vi "Checksum (SubVI).vi"(0 "StrIn":string="GPRMC,155547.000,A,0253.0515,S,07900.7371,W,0.00,,010113,,,A") -> (1 "Checksum":string, 2 "ChkSum":u8 format="%x")   [LabVIEW 2012]
doc: "moreChemistry's general purpose CRC vi\ncopyright 2004 moreChemistry BART BOSHUIZEN"
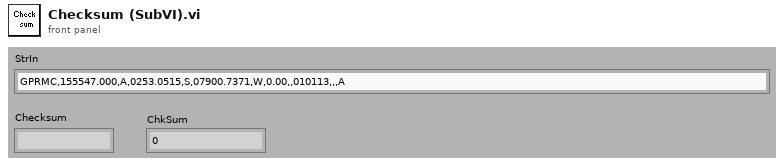
[diagram p1: front panel]
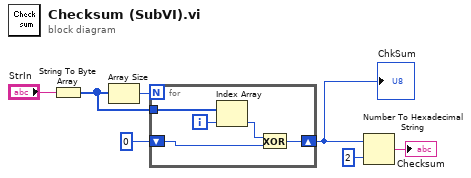
[diagram p0: block diagram]
diagram:
  n1 = String To Byte Array(string="StrIn") -> (unsigned byte array=w2:u8[])
  n2 = Array Size(array=w2) -> (size(s)=w5:i32)
  n3 = for {
    N: w5 -> [_]
    tunnel: w2 -> [w12]
    shift-right: [w10] -> w7
    shift-left: u8 0 -> [w9]
    i -> [w11]
    n4 = Index Array(array=w12, index=w11) -> (element=w8:u8)
    n5 = Exclusive Or(1:w9, 2:w8) -> (0:w10:u8)
  }
  "ChkSum" <- w7
  n6 = Number To Hexadecimal String(1:i16 2 ("width (-)"), 2:w7) -> (0:→"Checksum":string)
